vi "ActionVIOnLoad.vi"(8 "error in (no error)":errorcluster, 11 "Device Item Ref in":T1 format="%.0x") -> (0 "error out":errorcluster, 3 "Device Item Ref out":T1 format="%.0x")   [LabVIEW 2015, in "SLSC-12201 DIO System Explorer.lvlib"]
uses:
  SLSC-12201 DIO System Explorer.lvlib
  <vilib>/NI Veristand/Custom Device API/Custom Device Item Ref.ctl
  NationalInstruments.VeriStand.SystemDefinitionAPI
  Shared/Constants.vi
  <vilib>/NI Veristand/Custom Device Tools/Custom Device Utility Library/NI VeriStand - Search for All Items by Name.vi
  <vilib>/NI Veristand/Custom Device API/Custom Device API.lvlib
  Shared/SLSC-12201 DIO Shared.lvlib
  <vilib>/NI Veristand/Custom Device Tools/Custom Device Utility Library/Custom Device Utility Library.lvlib
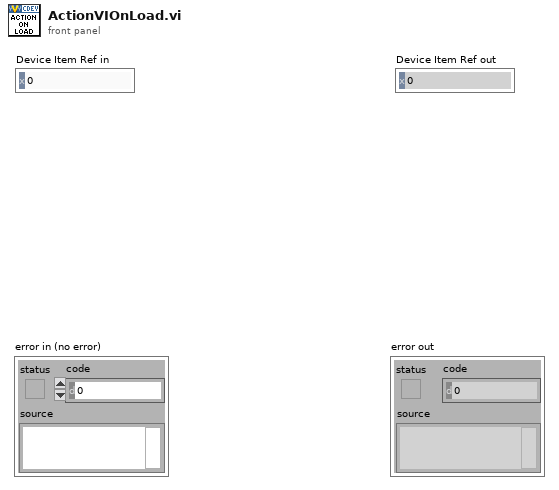
[diagram p1: front panel]
types:
  T1 = typedef "Custom Device API.lvlib/Custom Device Item Ref.ctl" = u64
  T2 = typedef "SLSC-12201 DIO System Explorer.lvlib/SLSC Channel Information.ctl" = cluster{"Channel Name":string, "SLSC Name":string, "Configuration":T3, "Enum Names":string[], "Enum Values":i32[]}
  T3 = typedef "Custom Device API.lvlib/Custom Device Channel.ctl" = cluster{"Type":T4, "Units":string, "Default Value":dbl, "Faultable":bool, "Scalable":bool}
  T4 = typedef "Custom Device API.lvlib/Custom Device Channel Type.ctl" = enum16{"Input", "Output"}
  T5 = cluster{"Channel Name":string, "SLSC Name":string, "Channel":T3, "Enum Names":string[], "Enum Values":i32[]}[]
  T6 = typedef "Custom Device API.lvlib/Custom Device Item Info.ctl" = cluster{"Name":string, "Is Channel":bool, "GUID":string, "Is Waveform":bool}
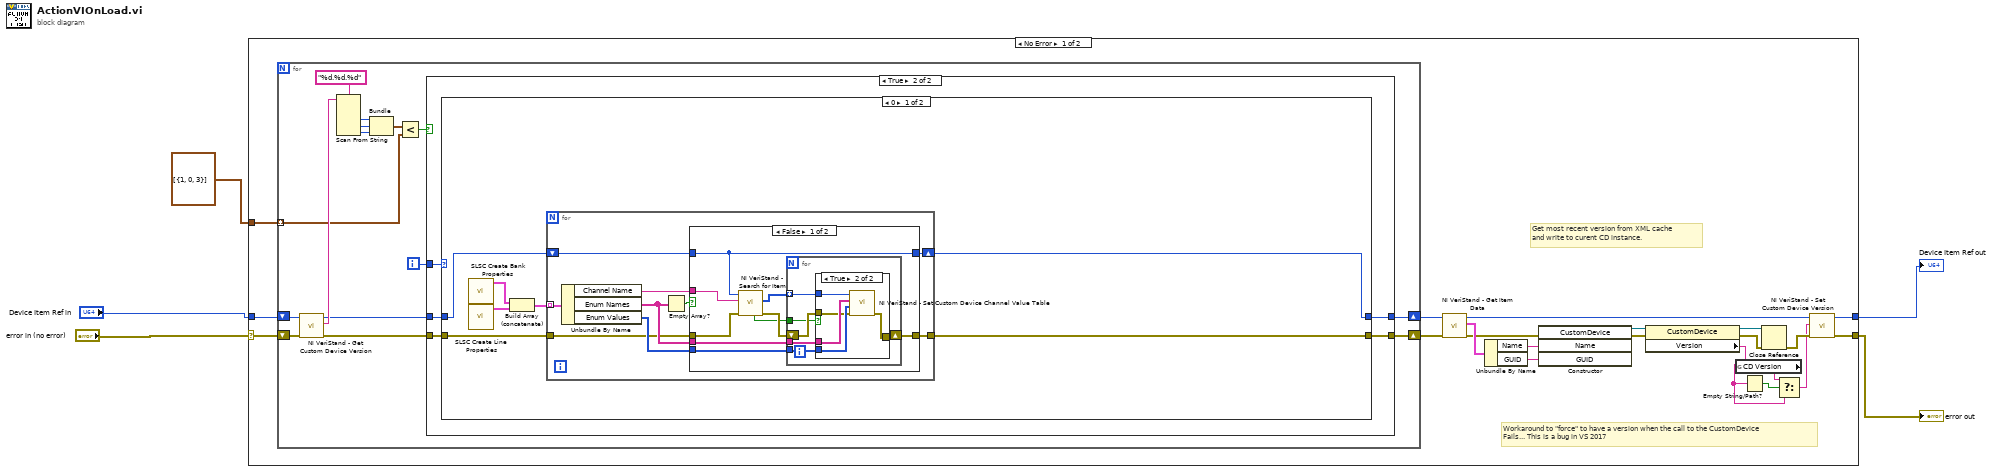
[diagram p0: block diagram]
diagram:
  n1 = case shown="No Error" "error in (no error)" {
    selector: "error in (no error)" -> [w26 w91]
    tunnel: [w10 w91] -> w2
    tunnel: "Device Item Ref in" -> [w25 w90]
    tunnel: [w11 w90] -> w3
    tunnel: cluster{i32, i32, i32}[] [{1, 0, 3}] -> [w24 _]
    frame No Error {
      # "Workaround to \"force\" to have a version when the call to the CustomDevice\nFails... This is a bug in VS 2017"
      # "Get most recent version from XML cache\nand write to curent CD instance."
      n2 = for {
        shift-right: [w32] -> w22
        shift-left: w26 -> [w37]
        shift-right: [w30] -> w23
        shift-left: w25 -> [w36]
        tunnel: w24 -> [w27] mode=indexing
        i -> [w29]
        n3 = call <vilib>:"NI VeriStand - Get Custom Device Version.vi"("error in (no error)"=w37, "Device Ref in"=w36) -> ("error out"=w33:errorcluster, "Value"=w35:string, "Device Ref out"=w31:T1)  [unwired: 7 in]
        n4 = Scan From String(format string="%d.%d.%d", input string=w35) -> (output 1=w39:i32, output 2=w40:i32, output 3=w28:i32)  [unwired: 5 in, 3 out]
        n5 = Bundle(w39, w40, w28) -> (w41:cluster{i32, i32, i32})  [unwired: 1 in]
        n6 = Less?(x=w41, y=w27) -> (x < y?=w34:bool)
        n7 = case shown="True" w34 {
          tunnel: w33 -> [w43 w48]
          tunnel: [w43 w47] -> w32
          tunnel: w31 -> [w42 w44]
          tunnel: [w42 w45] -> w30
          tunnel: w29 -> [_ w46]
          frame False {
          }
          frame True {
            n8 = case shown="0" w46 {
              tunnel: w48 -> [w53 w89]
              tunnel: [w52 w89] -> w47
              tunnel: [w49 w88] -> w45
              tunnel: w44 -> [w54 w88]
              frame 0 {
                n9 = call "SLSC Create Bank Properties.vi"() -> ("Outgoing configuration"=w55:T2[])  [unwired: 10 in, 1 out]
                n10 = call "SLSC Create Line Properties.vi"() -> ("Outgoing configuration"=w50:T5)  [unwired: 11 in]
                n11 = Build Array (concatenate)(w55, w50) -> (w51:T2[])
                n12 = for {
                  tunnel: w51 -> [w64] mode=indexing
                  tunnel: w53 -> [w58]
                  tunnel: [w57] -> w52
                  shift-right: [w56] -> w49
                  shift-left: w54 -> [w61]
                  n13 = Unbundle By Name(w64) -> ("Channel Name"=w63:string, "Enum Names"=w60:string[], "Enum Values"=w59:i32[])
                  n14 = Empty Array?(array=w60) -> (empty?=w62:bool)
                  n15 = case shown="False" w62 {
                    tunnel: w63 -> [w68 _]
                    tunnel: w61 -> [w65 w86]
                    tunnel: w60 -> [w73 _]
                    tunnel: w59 -> [w72 _]
                    tunnel: w58 -> [w71 w87]
                    tunnel: [w69 w87] -> w57
                    tunnel: [w65 w86] -> w56
                    frame False {
                      n16 = call-poly <vilib>:"NI VeriStand - Search for Item.vi"("error in"=w71, "Item Name"=w68, "Section Ref in"=w65) -> ("error out"=w70:errorcluster, "Item Refs"=w66:T1[], "Found"=w67:bool)  [unwired: 5 in, 1 out]
                      n17 = for {
                        tunnel: w73 -> [w79]
                        tunnel: w72 -> [w78]
                        tunnel: w67 -> [w75]
                        tunnel: w66 -> [w74] mode=indexing
                        shift-right: [w76] -> w69
                        shift-left: w70 -> [w77]
                        n18 = case shown="True" w75 {
                          tunnel: w74 -> [_ w85]
                          tunnel: w79 -> [_ w84]
                          tunnel: w78 -> [_ w83]
                          tunnel: w77 -> [w80 w82]
                          tunnel: [w80 w81] -> w76
                          frame False {
                          }
                          frame True {
                            n19 = call <vilib>:"NI VeriStand - Set Custom Device Channel Value Table.vi"("error in (no error)"=w82, "Values"=w83, "Names"=w84, "Channel Ref in"=w85) -> ("error out"=w81:errorcluster)  [unwired: 6 in, 1 out]
                          }
                        }
                      }
                    }
                    frame True {
                    }
                  }
                }
              }
              frame Default {
              }
            }
          }
        }
      }
      n20 = call <vilib>:"NI VeriStand - Get Item Data.vi"("error in (no error)"=w22, "Item Ref in"=w23) -> ("error out"=w18:errorcluster, "Item Info"=w21:T6, "Item Ref out"=w12:T1)  [unwired: 6 in, 1 out]
      n21 = Unbundle By Name(w21) -> ("Name"=w20:string, "GUID"=w19:string)
      n22 = constructor class="CustomDevice"(error in=w18, "Name"=w20, "GUID"=w19) -> (reference out=w17:refnum<k24>, error out=w16:errorcluster)  [unwired: 2 in, 3 out]
      n23 = property class="CustomDevice"(reference=w17, error in=w16) -> (reference out=w14:refnum<k24>, error out=w15:errorcluster, "Version"=w8:string)
      n24 = global read "Constants.vi" "CD Version"() -> (w7:string)
      n25 = Empty String/Path?(string/path=w8) -> (empty?=w9:bool)
      n26 = Close Reference(reference=w14, error in (no error)=w15) -> (error out=w13:errorcluster)
      n27 = Select(t=w7, s=w9, f=w8) -> (s? t:f=w6:string)
      n28 = call <vilib>:"NI VeriStand - Set Custom Device Version.vi"("error in (no error)"=w13, "Value"=w6, "Device Ref in"=w12) -> ("error out"=w10:errorcluster, "Device Ref out"=w11:T1)  [unwired: 7 in]
    }
    frame Error {
    }
  }
  "error out" <- w2
  "Device Item Ref out" <- w3
